vi "AutoInit.vi"(6 "D":dbl, 8 "I":dbl, 9 "P":dbl, 10 "Type":i32, 11 "ID":i32) -> (1 "Done?":bool)   [LabVIEW 2014]
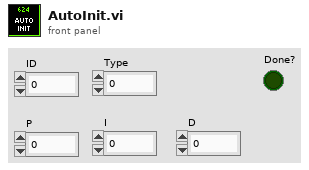
[diagram p1: front panel]
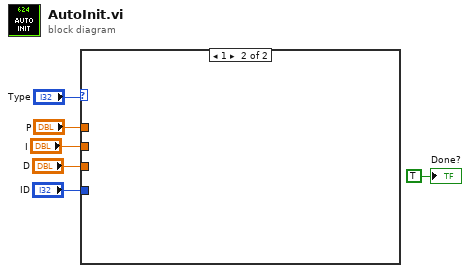
[diagram p0: block diagram]
diagram:
  n1 = case shown="1" "Type" {
    tunnel: "P" -> [w10 _]
    tunnel: "I" -> [w9 _]
    tunnel: "D" -> [w8 _]
    tunnel: "ID" -> [w7 _]
    frame 0, Default {
      n2 = case shown="0, Default" w7 {
        tunnel: w10 -> [_ _]
        tunnel: w9 -> [_ _]
        tunnel: w8 -> [_ _]
        frame 0, Default {
        }
        frame 1 {
        }
      }
    }
    frame 1 {
    }
  }
  "Done?" <- TRUE ("Done?")
